vi "Write Relay Map.vi"(8 "error in (no error)":errorcluster, 10 "Relay Map":i32[](array[numeric])=[97, 93, 89, 85, 81, 77, 73, 69, 65, 61, 57, 53, 47, 44, 40, 39, 32, 28, 24, 20, 16, 11, 7, 3, 52, 56, 60, 64, 68, 72, 76, 80, 84, 87, 91, 95, 2, 6, 10, 14, 19, 23, 27, 31, 35, 38, 43, 46, 96, 92, 88, 83, 79, 75, 71, 67, 63, 59, 55, 51, 45, 42, 37, 34, 30, 26, 22, 18, 13, 9, 5, 1, 50, 54, 58, 62, 66, 70, 74, 78, 82, 86, 90, 94, 0, 4, 8, 12, 17, 21, 25, 29, 33, 36, 41, 48, 49, 98], 11 "2575 in":refnum<class "2575.lvclass">) -> (0 "error out":errorcluster, 3 "2575 out":refnum<class "2575.lvclass">)   [LabVIEW 2019, in "2575.lvlib" / "2575.lvclass"]
uses:
  Library/2575.lvclass
  Library/2575.lvclass/2575.ctl
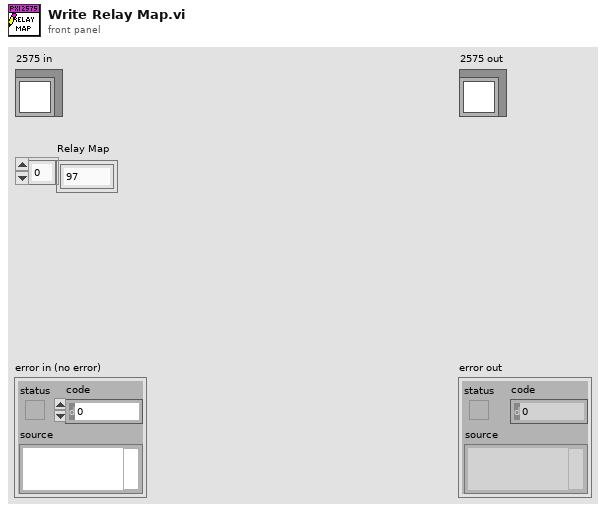
[diagram p1: front panel]
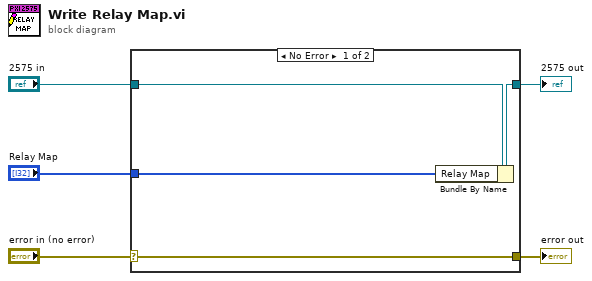
[diagram p0: block diagram]
diagram:
  n1 = case shown="No Error" "error in (no error)" {
    selector: "error in (no error)" -> [w9 w10]
    tunnel: [w9 w10] -> w4
    tunnel: [w7 w11] -> w2
    tunnel: "2575 in" -> [w8 w11]
    tunnel: "Relay Map" -> [w6 _]
    frame No Error {
      n2 = Bundle By Name(cluster=w8, "Relay Map"=w6) -> (w7:refnum<class "2575.lvclass">)
    }
    frame Error {
    }
  }
  "error out" <- w4
  "2575 out" <- w2
